vi "Release Session.vi"(0 "OBJ - Session in":refnum<class "niRFUtil Session.lvclass">, 5 "Session Handle in":T2, 11 "error in (no error)":errorcluster, 13 "Force Destroy? (F)":T1) -> (4 "OBJ - Session out":refnum<class "niRFUtil Session.lvclass">, 15 "error out":errorcluster)   [LabVIEW 2016, in "niRFUtil.lvlib" / "niRFUtil Session.lvclass"]
doc: "Initializes a measurement session\n\nSession data is set to the default values from \"set Defaults.vi\""
uses:
  niRFUtil Session.lvclass
  Includes/niRFUtil INC Session Handle.ctl
  Includes/niRFUtil INC Force Destroy.ctl
  niRFUtil.lvlib
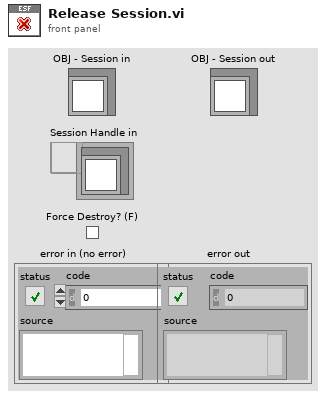
[diagram p1: front panel]
types:
  T1 = typedef "niRFUtil.lvlib/niRFUtil INC Force Destroy.ctl" = bool
  T2 = typedef "niRFUtil.lvlib/niRFUtil Session.lvclass/niRFUtil INC Session Handle.ctl" = refnum<data-value>
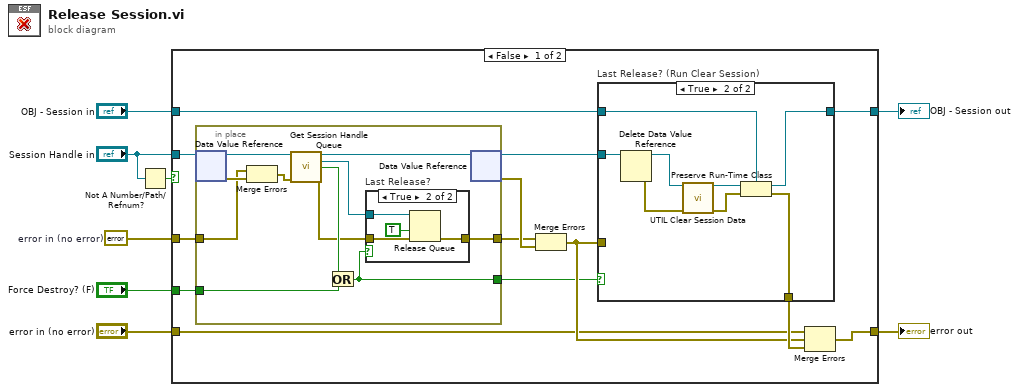
[diagram p0: block diagram]
diagram:
  w3 = errorcluster {"status"=FALSE, "code"=0, "source"=""}  # error in (no error)
  n1 = Not A Number/Path/Refnum?(number/path/refnum="Session Handle in") -> (NaN/Path/Refnum?=w1:bool)
  n2 = case shown="False" w1 {
    tunnel: "OBJ - Session in" -> [w21 w49]
    tunnel: [w20 w49] -> w7
    tunnel: "Session Handle in" -> [w19 _]
    tunnel: "Force Destroy? (F)" -> [w18 _]
    tunnel: [w14 w48] -> w5
    tunnel: "error in (no error)" -> [w12 w48]
    tunnel: w3 -> [w11 _]
    frame False {
      n3 = in-place {
        in-place-border: [w22] -> w9
        in-place-border: w18 -> [w24]
        in-place-border: w11 -> [w27]
        in-place-border: [w25] -> w10
        n4 = in-place-dvr #1(w19) -> (w32:refnum<class "niRFUtil Session.lvclass">, w29:errorcluster)
        n5 = Merge Errors(w27, w29) -> (w28:errorcluster)
        n6 = call "Get Session Handle Queue.vi"("OBJ - Session in"=w32, "error in (no error)"=w28) -> ("OBJ - Session out"=w31:refnum<class "niRFUtil Session.lvclass">, "Session Queue Handle"=w26:refnum<queue>, "Last Session?"=w30:bool, "error out"=w23:errorcluster)  [unwired: 10 in]
        n7 = Or(x=w30, y=w24) -> (x .or. y?=w22:T1)
        n8 = case "Last Release?" shown="True" w22 {
          tunnel: w26 -> [_ w37]
          tunnel: [w33 w36] -> w25
          tunnel: w23 -> [w33 w35]
          frame False {
          }
          frame True {
            n9 = Release Queue(queue=w37, force destroy? (F)=TRUE, error in (no error)=w35) -> (error out=w36:errorcluster)  [unwired: 2 out]
          }
        }
        n10 = in-place-dvr #1(w31) -> (w17:T2, w16:errorcluster)
      }
      n11 = Merge Errors(w10, w16) -> (w13:errorcluster)
      n12 = case "Last Release? (Run Clear Session)" shown="True" w9 {
        tunnel: w21 -> [w39 w45]
        tunnel: [w39 w42] -> w20
        tunnel: w17 -> [_ w47]
        tunnel: w13 -> [w38 _]
        tunnel: [w38 w40] -> w15
        frame False {
        }
        frame True {
          n13 = Delete Data Value Reference(data value reference=w47) -> (data value=w46:refnum<class "niRFUtil Session.lvclass">, error out=w41:errorcluster)  [unwired: 1 in]
          n14 = call-dynamic "UTIL Clear Session Data.vi"("OBJ - Measurement Session in"=w46, "error in"=w41) -> ("OBJ - Measurement Session out"=w43:refnum<class "niRFUtil Session.lvclass">, "error out"=w44:errorcluster)  [unwired: 12 in]
          n15 = Preserve Run-Time Class(object in=w43, error in=w44, 2:w45) -> (object out=w42:refnum<class "niRFUtil Session.lvclass">, error out=w40:errorcluster)
        }
      }
      n16 = Merge Errors(w12, w13, w15) -> (w14:errorcluster)
    }
    frame True {
    }
  }
  "error out" <- w5
  "OBJ - Session out" <- w7
